vi "Error Handler.vi"(8 "Error In":errorcluster, 9 "refnum in":refnum<file>) -> (0 "Error Out":errorcluster, 1 "refnum out":refnum<file>)   [LabVIEW 2020, in "Test Framework.lvclass"]
doc: "Error wrapper for the Test Framework class"
uses:
  Test Framework.lvclass
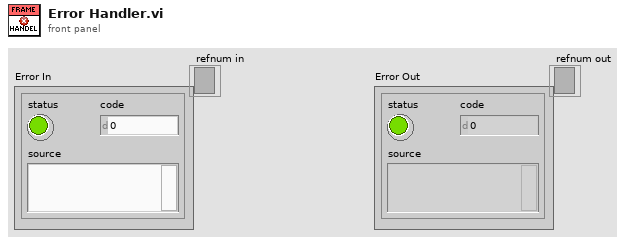
[diagram p1: front panel]
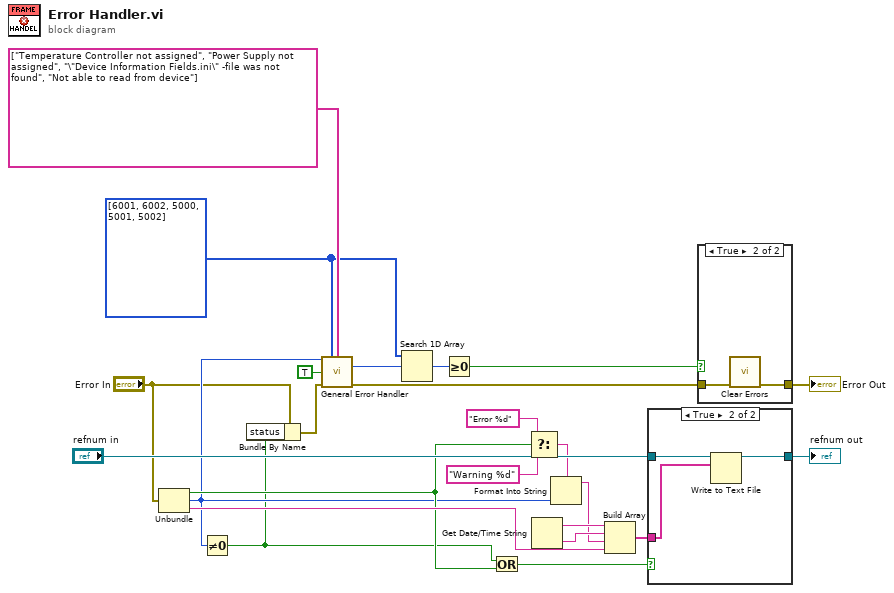
[diagram p0: block diagram]
diagram:
  w23 = i32[] [6001, 6002, 5000, 5001, 5002] ("[user-defined codes]")
  n1 = Unbundle("Error In") -> ("status"=w6:bool, "code"=w4:i32, "source"=w12:string)
  n2 = Not Equal To 0?(x=w4) -> (x != 0?=w3:bool)
  n3 = Bundle By Name(cluster="Error In", "status"=w3) -> (w1:errorcluster)
  n4 = call <vilib>:"General Error Handler.vi"("[error code] (0)"=w4, "[user-defined codes]"=w23, "[user-defined descriptions]"=string[] ["Temperature Controller not assigned", "Power Supply not assigned", "\"Device Information Fields.ini\" -file was not found", "Not able to read from device"], "search ni.com link visible?(T)"=TRUE, "error in (no error)"=w1) -> ("code out"=w22:i32, "error out"=w16:errorcluster)  [unwired: 6 in, 3 out]
  n5 = Search 1D Array(1D array=w23, element=w22) -> (index of element=w21:i32)  [unwired: 1 in]
  n6 = Greater Or Equal To 0?(x=w21) -> (x >= 0?=w20:bool)
  n7 = Or(x=w3, y=w6) -> (x .or. y?=w7:bool)
  n8 = Select(t="Error %d" ("format string"), s=w6, f="Warning %d" ("format string")) -> (s? t:f=w10:string)
  n9 = Get Date/Time String() -> (date string=w15:string, time string=w14:string)  [unwired: 3 in]
  n10 = Format Into String(format string=w10, w4) -> (resulting string=w13:string)  [unwired: 2 in, 1 out]
  n11 = Build Array(w15, w14, w13, w12) -> (w11:string[])
  n12 = case shown="True" w7 {
    tunnel: [w25 w28] -> w18
    tunnel: "refnum in" -> [w25 w27]
    tunnel: w11 -> [_ w26]
    frame False {
    }
    frame True {
      n13 = Write to Text File(file (use dialog)=w27, text=w26) -> (refnum out=w28:refnum<file>)  [unwired: 2 in, 2 out]
    }
  }
  "refnum out" <- w18
  n14 = case shown="True" w20 {
    tunnel: w16 -> [w29 w31]
    tunnel: [w29 w30] -> w19
    frame False {
    }
    frame True {
      n15 = call <vilib>:"Clear Errors.vi"("error in (no error)"=w31) -> ("error out"=w30:errorcluster)  [unwired: 5 in, 1 out]
    }
  }
  "Error Out" <- w19
